vi "gráfico_atv_VE.vi"() -> ()   [LabVIEW 2019]
uses:
  <vilib>/measure/matone.llb/Extract Multiple Tone Information N Chan.vi
  <vilib>/measure/NI_MAPro.lvlib
panel:
  out "multiple tone information":T1(array[cluster]) {"multiple tone information"."detected phase (deg)" format="%_6g"; "multiple tone information"."detected amplitude" format="%_6p"; "multiple tone information"."detected frequency" format="%_6p"}
  out "Waveform Graph":waveform(dbl)[](graph)
  in  "file path":path
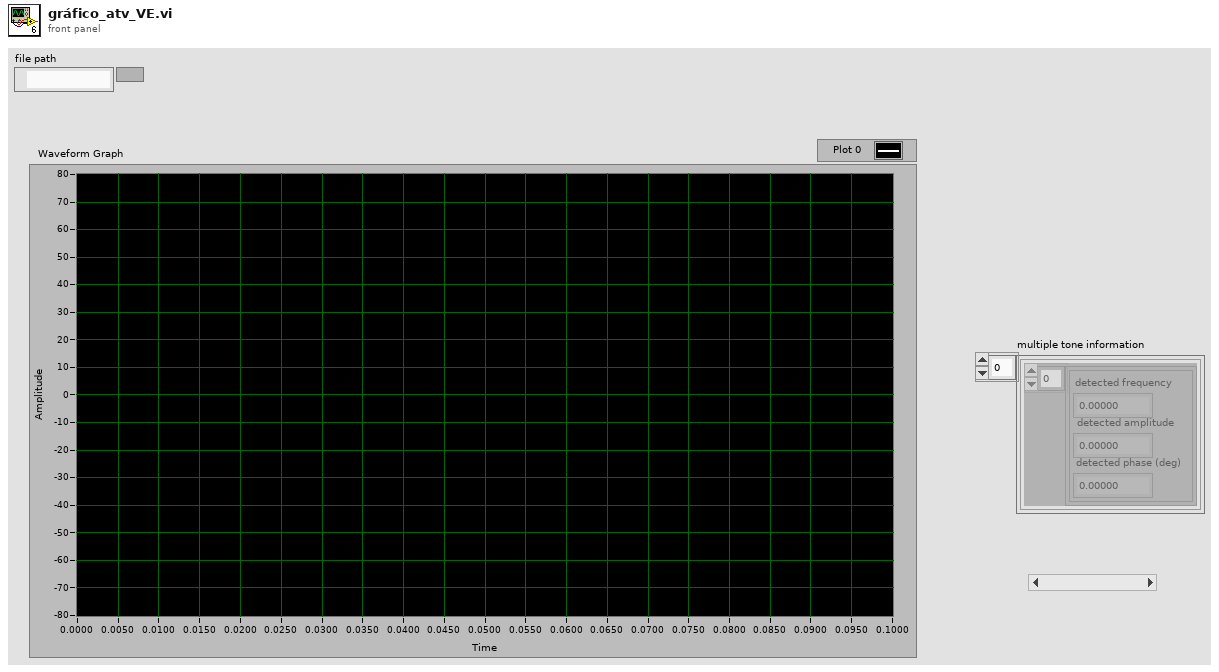
[diagram p1: front panel]
types:
  T1 = cluster{"multiple tone information":cluster{"detected frequency":dbl, "detected amplitude":dbl, "detected phase (deg)":dbl}[]}[]
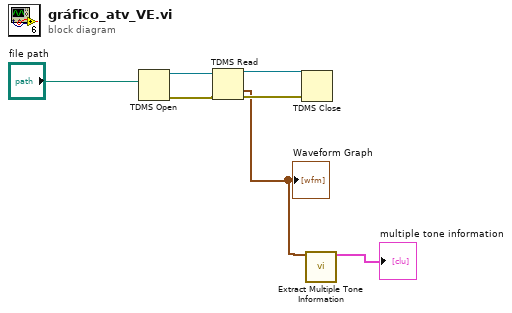
[diagram p0: block diagram]
diagram:
  n1 = TDMS Open(11:"file path") -> (0:w6:errorcluster, 3:w7:refnum<k34>)  [unwired: 6 in]
  n2 = TDMS Read(0:w7, 11:w6) -> (4:w5:refnum<k34>, 10:w2:waveform(dbl)[], 15:w4:errorcluster)  [unwired: 6 in, 3 out]
  "Waveform Graph" <- w2
  n3 = TDMS Close(8:w4, 11:w5) -> ()  [unwired: 2 out]
  n4 = call-poly <vilib>:"Extract Multiple Tone Information.vi"("time signals in"=w2) -> ("multiple tone information"=→"multiple tone information":T1)  [unwired: 12 in, 2 out]
